vi "Create C-string pointer.vi"(8 "error in (no error)":errorcluster, 11 "string":string) -> (0 "error out":errorcluster, 1 "size":i32, 2 "C-string pointer":i64, 3 "string out":string)   [LabVIEW 2013, in "SQLiteSupport.lvlib"]
uses:
  SQLiteSupport.lvlib
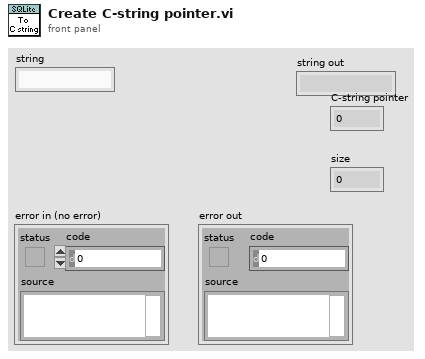
[diagram p1: front panel]
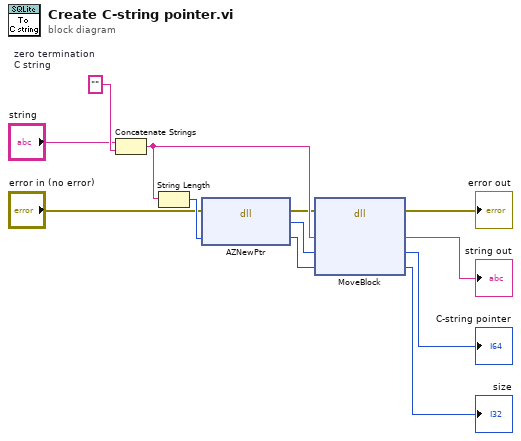
[diagram p0: block diagram]
diagram:
  w4 = ""  # zero termination C string
  n1 = Concatenate Strings("string", w4) -> (w12:string)
  n2 = String Length(string=w12) -> (length=w11:i32)
  n3 = dll-call lib="LabVIEW" fn="AZNewPtr"(error in="error in (no error)", "size"=w11) -> (error out=w8:errorcluster, "new pointer"=w2:i64, "size"=w3:i32)  [unwired: 2 in, 1 out]
  n4 = dll-call lib="LabVIEW" fn="MoveBlock"(error in=w8, "source"=w12, "destination"=w2, "size"=w3) -> (error out=→"error out":errorcluster, "source"=→"string out":string, "destination"=→"C-string pointer":i64, "size"=→"size":i32)  [unwired: 3 in, 1 out]
